vi "Main Module.vi"(8 "Error In":errorcluster) -> (0 "Error Out":errorcluster)   [LabVIEW 2015, in "Controller.lvlib"]
uses:
  Controller.lvlib
  Private Controls/Module Data Cluster.ctl
  Private Controls/Module Action.ctl
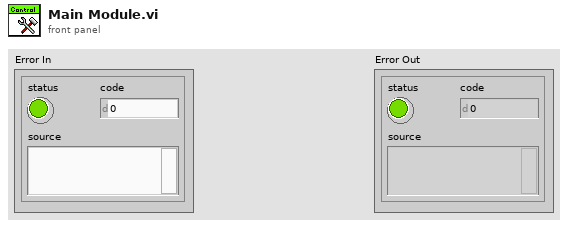
[diagram p1: front panel]
types:
  T1 = typedef "Controller.lvlib/Module Data Cluster.ctl" = cluster{"Data":variant, "Action":T2}
  T2 = typedef "Controller.lvlib/Module Action.ctl" = enum16{"Init", "Close", "Error", "Start Wash Operation"}
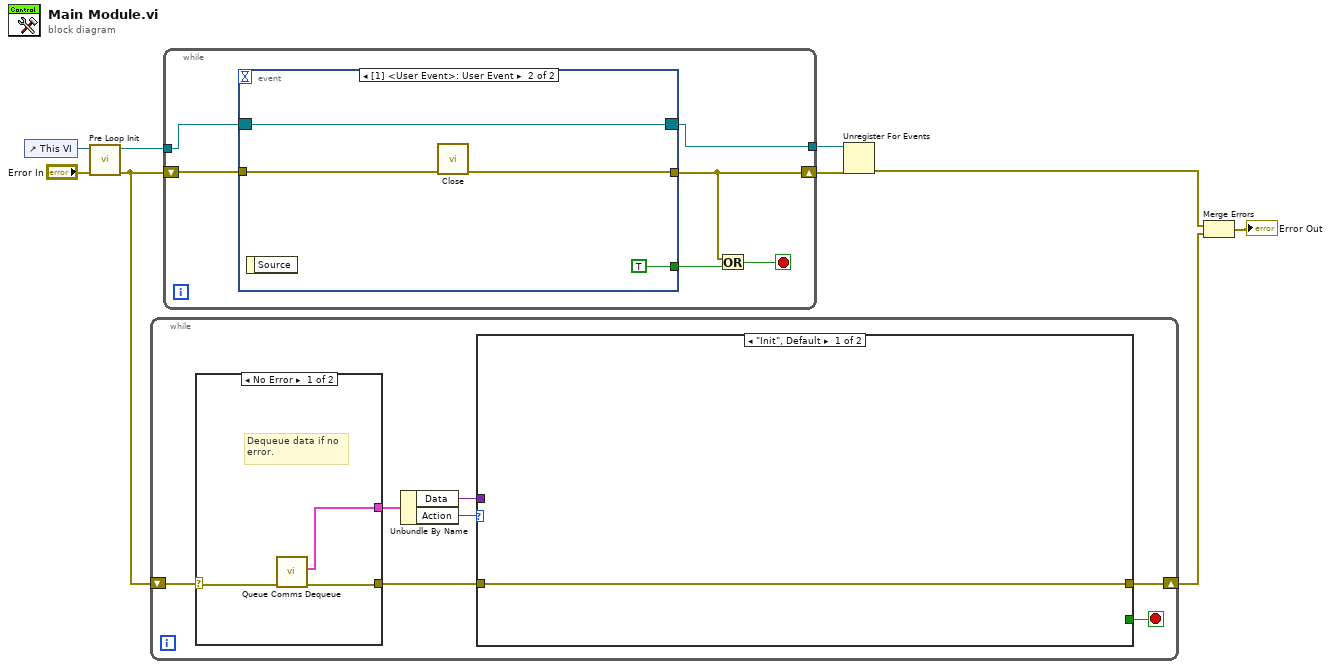
[diagram p0: block diagram]
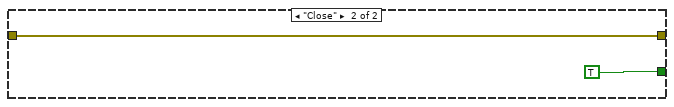
[diagram p2: hidden frame]
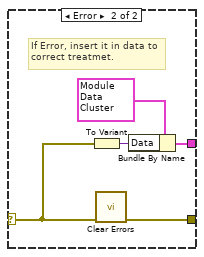
[diagram p3: hidden frame]
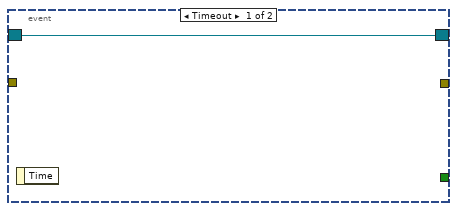
[diagram p4: hidden frame]
diagram:
  n1 = control-ref of="This VI"() -> (w8:refnum<vi>)
  n2 = call "Pre Loop Init.vi"("Error In"="Error In", "This VI"=w8) -> ("Error Out"=w4:errorcluster, "Event Registration Refnum"=w7:refnum<event-registration>)  [unwired: 8 in]
  n3 = while {
    shift-right: [w10] -> w2
    shift-left: w4 -> [w16]
    stop <- w11 stop-if-true
    n4 = case shown="No Error" w16 {
      selector: w16 -> [w22 w25]
      tunnel: [w21 w24] -> w13
      tunnel: [w20 w23] -> w15
      frame No Error {
        # "Dequeue data if no\nerror."
        n5 = call "Queue Comms Dequeue.vi"("Error In"=w22) -> ("Error Out"=w21:errorcluster, "Message Data"=w20:T1)  [unwired: 9 in]
      }
      frame Error {
        # "If Error, insert it in data to\ncorrect treatmet."
        n6 = To Variant(anything=w25) -> (Variant=w26:variant)
        n7 = call <vilib>:"Clear Errors.vi"("error in (no error)"=w25) -> ("error out"=w24:errorcluster)  [unwired: 5 in, 1 out]
        n8 = Bundle By Name(cluster=T1 {"Data"=variant, "Action"=enum."Error"} ("Message Data"), "Data"=w26) -> (w23:T1)
      }
    }
    n9 = Unbundle By Name(w15) -> ("Data"=w12:variant, "Action"=w14:T2)
    n10 = case shown="\"Init\", Default" w14 {
      tunnel: w13 -> [w17 w18]
      tunnel: w12 -> [_ _]
      tunnel: [_ TRUE] -> w11
      tunnel: [w17 w18] -> w10
      frame "Init", Default {
      }
      frame "Close" {
      }
    }
  }
  n11 = while {
    tunnel: w7 -> [w33]
    shift-right: [w30] -> w6
    shift-left: w4 -> [w31]
    tunnel: [w28] -> w5
    stop <- w32 stop-if-true
    n12 = event shown="[1] <User Event>: User Event" {
      selector: w33 -> [w34 w38]
      dyn-events: [w34 w38] -> w28
      timeout: _ -> [_ _]
      tunnel: [_ w36] -> w30
      tunnel: w31 -> [_ w37]
      tunnel: [_ TRUE] -> w29
      event Timeout {
        n13 = event-data() -> ()  [unwired: 1 in, 1 out]
      }
      event User Event {
        n14 = event-data() -> ()  [unwired: 1 in, 1 out]
        n15 = call "Close.vi"("Error In"=w37) -> ("Error Out"=w36:errorcluster)  [unwired: 10 in]
      }
    }
    n16 = Or(x=w30, y=w29) -> (x .or. y?=w32:bool)
  }
  n17 = Unregister For Events(event registration refnum=w5, error in=w6) -> (error out=w1:errorcluster)
  n18 = Merge Errors(w1, w2) -> (→"Error Out":errorcluster)
